vi "hw3p6_hickey.vi"() -> ()   [LabVIEW 2014]
panel:
  in  "Mu":dbl
  out "Waveform Graph":cluster{dbl, dbl, dbl[]}(graph)
  out "Array":dbl[](array[numeric])
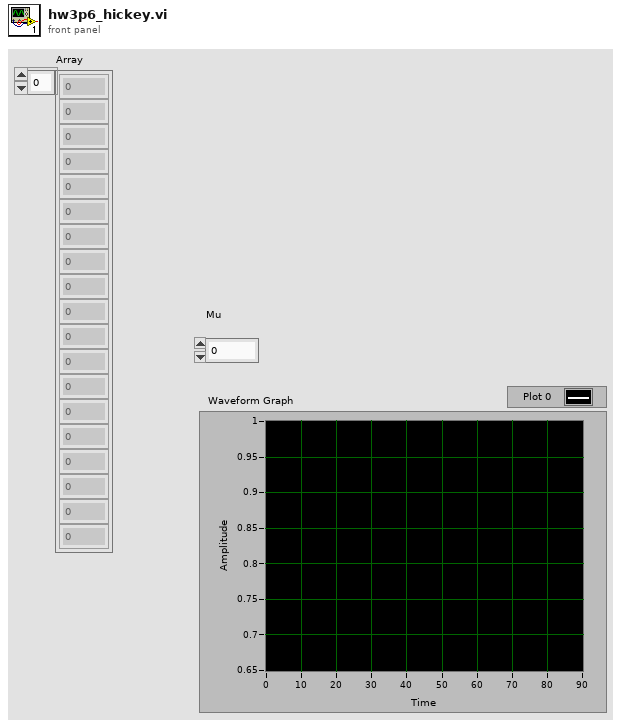
[diagram p1: front panel]
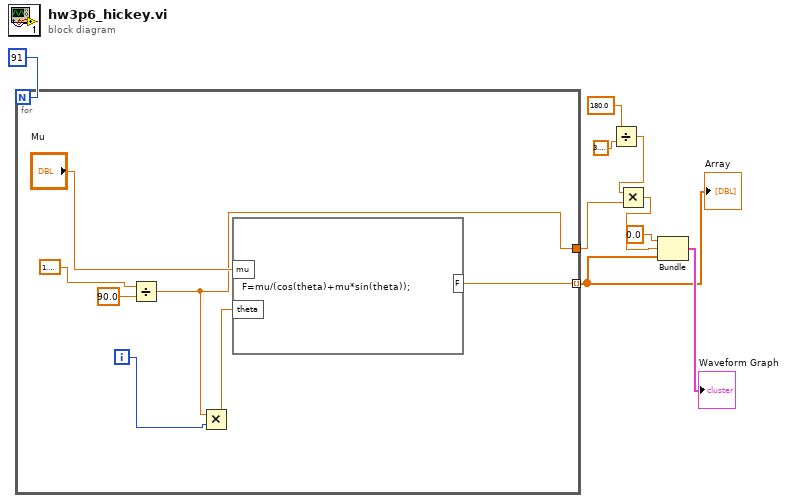
[diagram p0: block diagram]
diagram:
  n1 = for {
    N: 91 -> [_]
    tunnel: [w11] -> w6 mode=indexing
    tunnel: [w10] -> w2
    i -> [w13]
    n2 = Divide(x=1.5707963267948966, y=90.0) -> (x/y=w10:dbl)
    n3 = Multiply(x=w10, y=w13) -> (x*y=w12:dbl)
    n4 = formula code="F=mu/(cos(theta)+mu*sin(theta));"("mu"="Mu", "theta"=w12) -> ("F"=w11:dbl)
  }
  "Array" <- w6
  n5 = Divide(x=180.0, y=3.141592653589793) -> (x/y=w3:dbl)
  n6 = Multiply(x=w3, y=w2) -> (x*y=w1:dbl)
  n7 = Bundle(0.0, w1, w6) -> (→"Waveform Graph":cluster{dbl, dbl, dbl[]})  [unwired: 1 in]
